vi "Power Grad Read Array.vi"(8 "error in":errorcluster, 11 "Cycler in":refnum<class "Cycler.lvclass">) -> (0 "error out":errorcluster, 1 "Changed or First Call?":bool, 2 "Power SP":dbl[](array[numeric]), 3 "Cycler out":refnum<class "Cycler.lvclass">)   [LabVIEW 2023, in "Cycler.lvclass"]
uses:
  Cycler.lvclass
  Cycler.lvclass/Cycler.ctl
  Low Level Capabilities/Power/Power Gradient/Power Gradient.lvclass
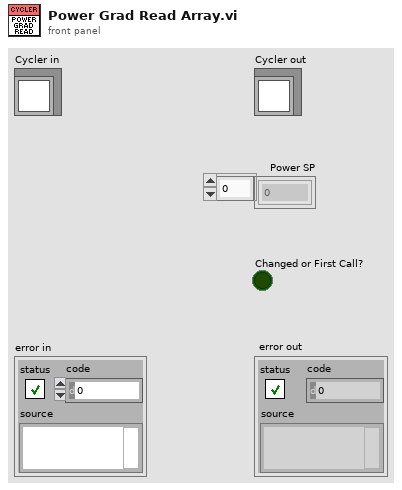
[diagram p1: front panel]
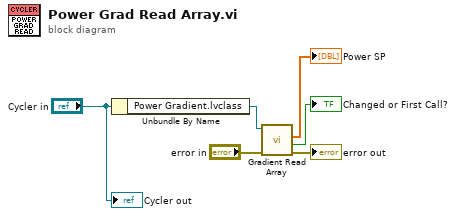
[diagram p0: block diagram]
diagram:
  n1 = Unbundle By Name("Cycler in") -> ("Power Gradient.lvclass"=w6:refnum<class "Power Gradient.lvclass">)
  n2 = call-dynamic "Gradient Read Array.vi"("error in"="error in", "Power Gradient in"=w6) -> ("error out"=→"error out":errorcluster, "Changed or First Call?"=→"Changed or First Call?":bool, "Power SP"=→"Power SP":dbl[])  [unwired: 6 in, 1 out]
  "Cycler out" <- "Cycler in"
